vi "Create Tx Word Description.vi"(8 "error in (no error)":errorcluster, 11 "Initial Value":u32) -> (0 "error out":errorcluster, 3 "Description":string)   [LabVIEW 2019, in "Ballard Arinc-429 System Explorer.lvlib"]
uses:
  Ballard Arinc-429 System Explorer.lvlib
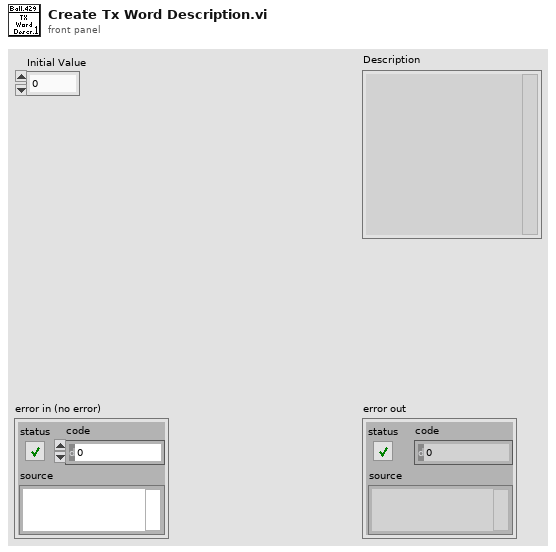
[diagram p1: front panel]
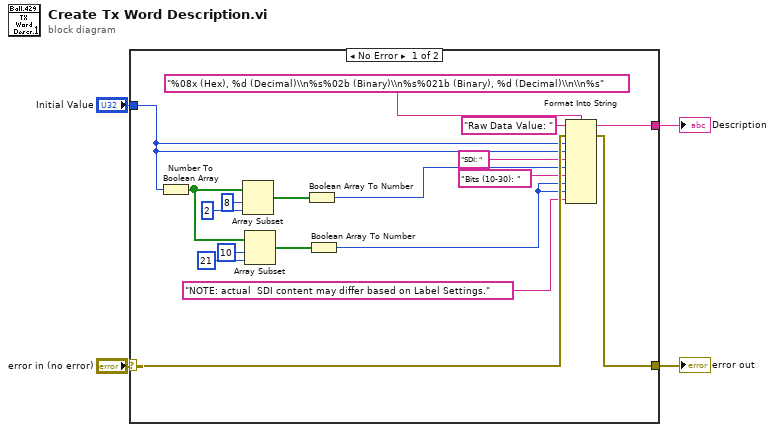
[diagram p0: block diagram]
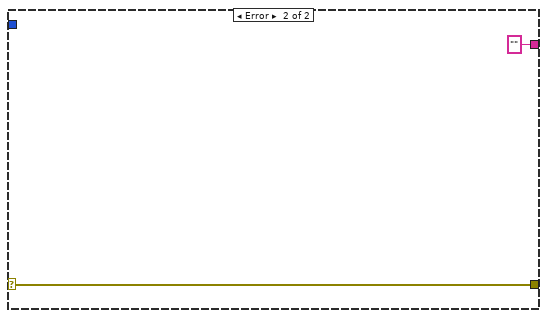
[diagram p2: hidden frame]
diagram:
  n1 = case shown="No Error" "error in (no error)" {
    selector: "error in (no error)" -> [w20 w24]
    tunnel: [w19 w24] -> w3
    tunnel: "Initial Value" -> [w15 _]
    tunnel: [w18 ""] -> w1
    frame No Error {
      n2 = Number To Boolean Array(number=w15) -> (Boolean array=w7:bool[])
      n3 = Array Subset(array=w7, index=8, length=2) -> (w13:bool[])
      n4 = Array Subset(array=w7, index=10, length=21) -> (w10:bool[])
      n5 = Boolean Array To Number(Boolean array=w13) -> (number=w12:u32)
      n6 = Boolean Array To Number(Boolean array=w10) -> (number=w6:u32)
      n7 = Format Into String(format string="%08x (Hex), %d (Decimal)\\n%s%02b (Binary)\\n%s%021b (Binary), %d (Decimal)\\n\\n%s", initial string="Raw Data Value: ", error in=w20, w15, w15, "SDI: " ("input 3"), w12, "Bits (10-30): " ("input 3"), w6, w6, "NOTE: actual  SDI content may differ based on Label Settings." ("input 8")) -> (resulting string=w18:string, error out=w19:errorcluster)
    }
    frame Error {
    }
  }
  "error out" <- w3
  "Description" <- w1
